vi "Polygon Intersection_Cross Product.vi"(8 "y 2":dbl, 9 "x 2":dbl, 10 "y 1":dbl, 11 "x 1":dbl) -> (3 "Corss Product":dbl)   [LabVIEW 2020, in "NI_AAL_Geometry.lvlib"]
uses:
  <vilib>/Analysis/NI_AAL_Geometry.lvlib
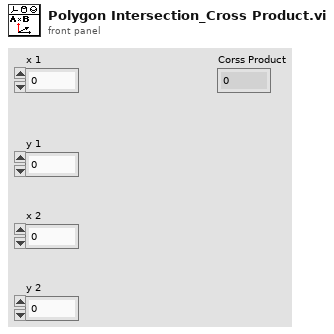
[diagram p1: front panel]
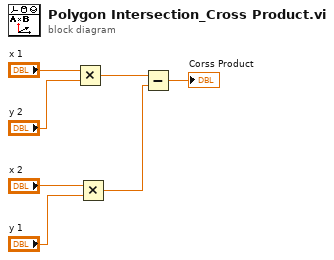
[diagram p0: block diagram]
diagram:
  n1 = Multiply(x="x 1", y="y 2") -> (x*y=w3:dbl)
  n2 = Multiply(x="x 2", y="y 1") -> (x*y=w2:dbl)
  n3 = Subtract(x=w3, y=w2) -> (x-y=→"Corss Product":dbl)
